vi "Heater_Safety.vi"   [LabVIEW 2010]
types:
  T1 = typedef "Ch_description_ADAM.ctl" = cluster{"Ch Name":string, "Type":T2, "Function":T3, "Ch State":T4, "Calibration type":T5, "A":dbl, "B":dbl, "C":dbl, "D":dbl, "Comments":string, "Address":T6, "String":string, "Duty":u16}
  T2 = typedef "Module_type_ADAM.ctl" = enum16{"4011", "4012", "4013", "4014", "4016", "4017", "4018", "4021", "4050", "4052", "4053", "4060", "4080", "5000", "5017", "5018", "5024", "5051", "5056", "5060", "6060", "Tracker", "WEST", "GILL", "JEM", "VICI", "Vaisala", "DRUCK", "Run VI Named:", "IR2100", "PPT", "Comparator", "VIRTUAL", "Hold Value", "Read A", "Read Ch", "Coded", "Client Info", "Web Client", "X10", "Test"}
  T3 = typedef "Function_ADAM.ctl" = enum16{"Analogue Input", "Digital Input", "Event counter", "Event rate", "Analogue Output", "Digital Output", "Relay Output"}
  T4 = typedef "Channel_State.ctl" = enum16{"On", "Off", "Always On", "Always Off"}
  T5 = typedef "Calib_type_ADAM.ctl" = enum16{"Raw", "Bx + A", "Cx^2 + Bx + A", "Dx^3 + Cx^2 + Bx + A", "In Band", "Hi-Tec Q", "Hi-Tec M_dot", "Text"}
  T6 = typedef "Address.ctl" = cluster{"Main":i32, "Ch.":i32, "Sub":i32, "Port Name":string}
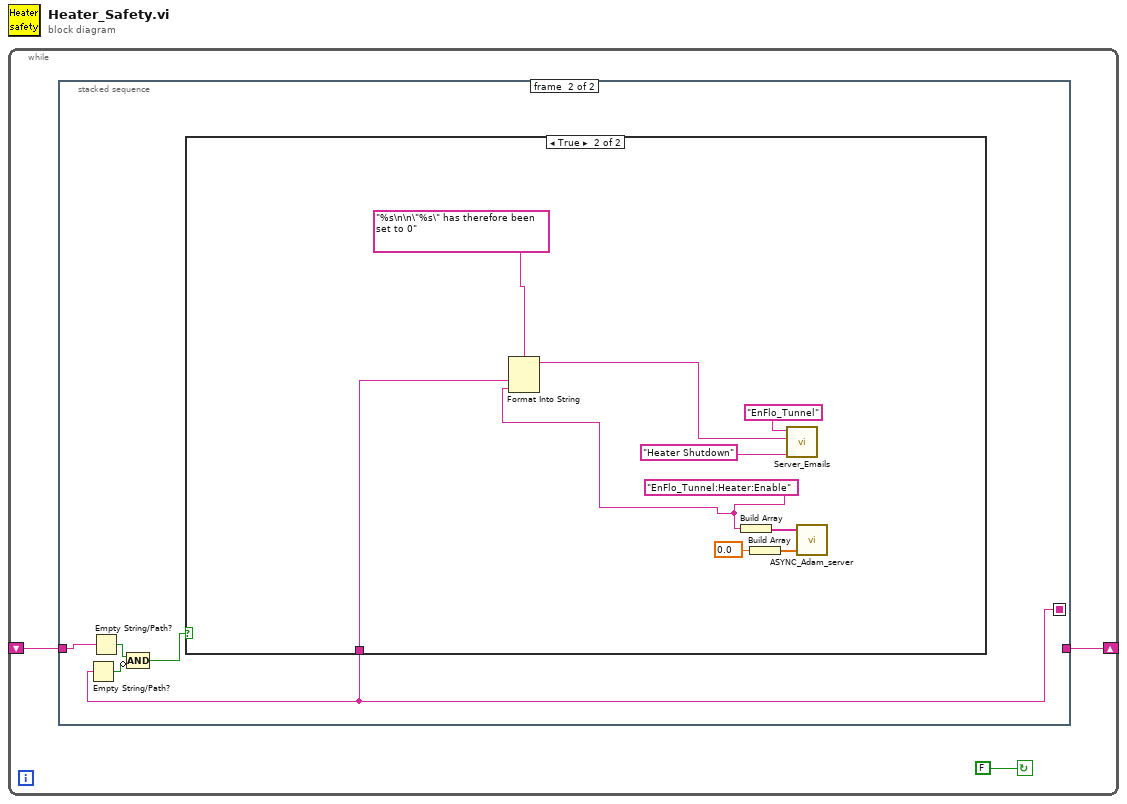
[diagram p0: block diagram]
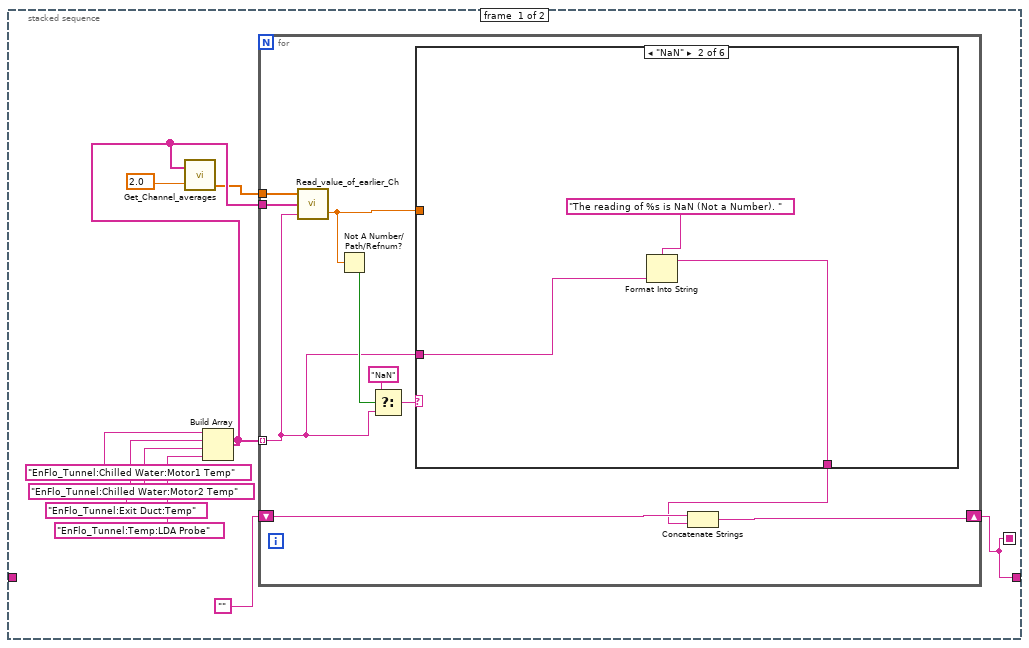
[diagram p2: hidden frame]
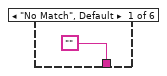
[diagram p3: hidden frame]
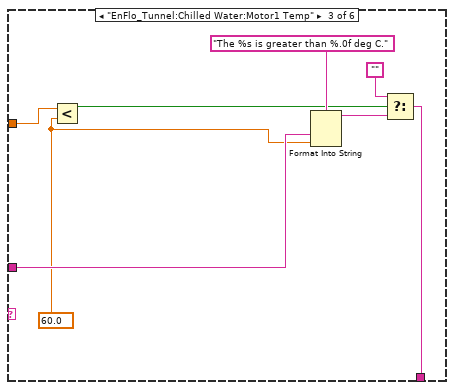
[diagram p4: hidden frame]
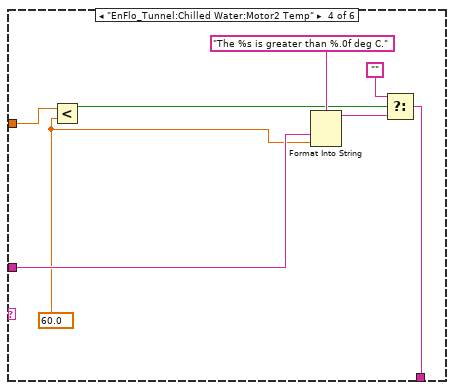
[diagram p5: hidden frame]
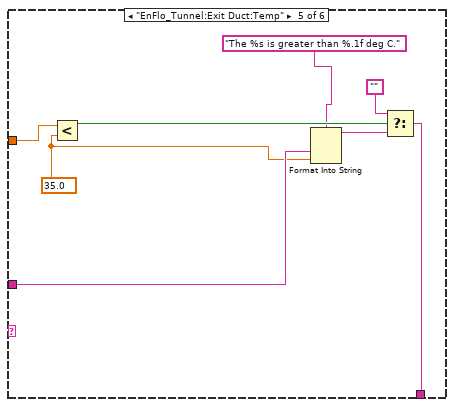
[diagram p6: hidden frame]
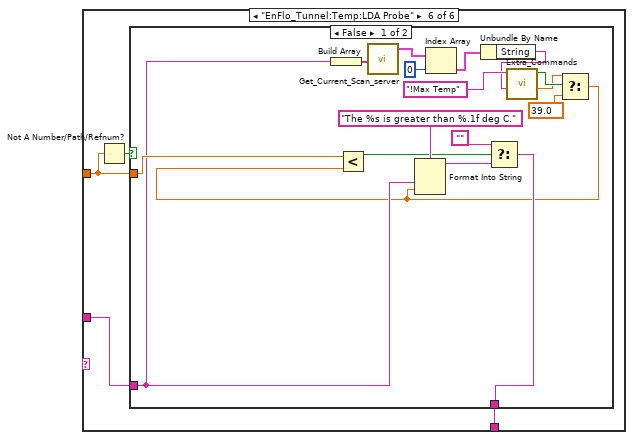
[diagram p7: hidden frame]
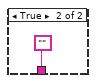
[diagram p8: hidden frame]
diagram:
  n1 = while {
    shift-left: _ -> [w1]
    shift-right: [w2] -> _
    stop <- FALSE continue-if-true
    n2 = stacked-sequence {
      seq-local: [w5 _] -> [_ w73]
      tunnel: [w5 _] -> w2
      tunnel: w1 -> [_ w77]
      frame #0 {
        n3 = Build Array("EnFlo_Tunnel:Chilled Water:Motor1 Temp", "EnFlo_Tunnel:Chilled Water:Motor2 Temp", "EnFlo_Tunnel:Exit Duct:Temp", "EnFlo_Tunnel:Temp:LDA Probe") -> (w9:string[])
        n4 = call "Get_Channel_averages.vi"("Desired Ch Names"=w9, "Averaging time (mins)"=2.0) -> ("number"=w6:dbl[])  [unwired: 1 in, 2 out]
        n5 = for {
          tunnel: w9 -> [w21]
          tunnel: w6 -> [w22]
          tunnel: w9 -> [w14] mode=indexing
          shift-right: [w19] -> w5
          shift-left: "" -> [w20]
          n6 = call "Read_value_of_earlier_Ch.vi"("Desired Ch to Read"=w14, "Ch names"=w21, "Present scan array"=w22) -> ("Value"=w17:dbl)  [unwired: 1 in, 1 out]
          n7 = Not A Number/Path/Refnum?(number/path/refnum=w17) -> (NaN/Path/Refnum?=w16:bool)
          n8 = Select(t="NaN", s=w16, f=w14) -> (s? t:f=w13:string)
          n9 = case shown="\"NaN\"" w13 {
            tunnel: w17 -> [_ _ w34 w42 w46 w52]
            tunnel: w14 -> [_ w24 w33 w41 w50 w54]
            tunnel: ["" w25 w27 w35 w47 w53] -> w18
            frame "No Match", Default {
            }
            frame "NaN" {
              n10 = Format Into String(format string="The reading of %s is NaN (Not a Number). " ("Format String"), w24) -> (resulting string=w25:string)  [unwired: 2 in, 1 out]
            }
            frame "EnFlo_Tunnel:Chilled Water:Motor1 Temp" {
              w32 = 60.0 ("y")
              n11 = Less?(x=w34, y=w32) -> (x < y?=w30:bool)
              n12 = Format Into String(format string="The %s is greater than %.0f deg C." ("Format String"), w33, w32) -> (resulting string=w29:string)  [unwired: 2 in, 1 out]
              n13 = Select(t="", s=w30, f=w29) -> (s? t:f=w27:string)
            }
            frame "EnFlo_Tunnel:Chilled Water:Motor2 Temp" {
              w40 = 60.0 ("y")
              n14 = Less?(x=w42, y=w40) -> (x < y?=w38:bool)
              n15 = Format Into String(format string="The %s is greater than %.0f deg C." ("Format String"), w41, w40) -> (resulting string=w37:string)  [unwired: 2 in, 1 out]
              n16 = Select(t="", s=w38, f=w37) -> (s? t:f=w35:string)
            }
            frame "EnFlo_Tunnel:Exit Duct:Temp" {
              w49 = 35.0 ("y")
              n17 = Less?(x=w46, y=w49) -> (x < y?=w48:bool)
              n18 = Format Into String(format string="The %s is greater than %.1f deg C." ("Format String"), w50, w49) -> (resulting string=w44:string)  [unwired: 2 in, 1 out]
              n19 = Select(t="", s=w48, f=w44) -> (s? t:f=w47:string)
            }
            frame "EnFlo_Tunnel:Temp:LDA Probe" {
              n20 = Not A Number/Path/Refnum?(number/path/refnum=w52) -> (NaN/Path/Refnum?=w51:bool)
              n21 = case shown="False" w51 {
                tunnel: w52 -> [w71 _]
                tunnel: w54 -> [w65 _]
                tunnel: [w66 ""] -> w53
                frame False {
                  n22 = Build Array(w65) -> (w64:string[])
                  n23 = call "Get_Current_Scan_server.vi"("Desired Channels"=w64) -> ("Ch Description Array"=w63:T1[])  [unwired: 2 out]
                  n24 = Index Array(array=w63, index=0 ("Index")) -> (element=w61:T1)
                  n25 = Unbundle By Name(w61) -> ("String"=w55:string)
                  n26 = call "Extra_Commands.vi"("String to Search"=w55, "Command"="!Max Temp") -> ("Numeric Value"=w58:dbl, "Command Found"=w59:bool)  [unwired: 1 in, 3 out]
                  n27 = Select(t=w58, s=w59, f=39.0) -> (s? t:f=w56:dbl)
                  n28 = Less?(x=w71, y=w56) -> (x < y?=w67:bool)
                  n29 = Format Into String(format string="The %s is greater than %.1f deg C." ("Format String"), w65, w56) -> (resulting string=w69:string)  [unwired: 2 in, 1 out]
                  n30 = Select(t="", s=w67, f=w69) -> (s? t:f=w66:string)
                }
                frame True {
                }
              }
            }
          }
          n31 = Concatenate Strings(w20, w18) -> (w19:string)
        }
      }
      frame #1 {
        n32 = Empty String/Path?(string/path=w73) -> (empty?=w75:bool)
        n33 = Empty String/Path?(string/path=w77) -> (empty?=w76:bool)
        n34 = Compound Arithmetic op=AND(w76, invert w75) -> (w74:bool)
        n35 = case shown="True" w74 {
          tunnel: w73 -> [_ w79]
          frame False {
          }
          frame True {
            w80 = "EnFlo_Tunnel:Heater:Enable"
            n36 = Format Into String(format string="%s\n\n\"%s\" has therefore been set to 0", w79, w80) -> (resulting string=w78:string)  [unwired: 2 in, 1 out]
            n37 = Build Array(w80) -> (w81:string[])
            n38 = Build Array(0.0) -> (w82:dbl[])
            n39 = call "Server_Emails.vi"("Client Name Contains"="EnFlo_Tunnel", "Message"=w78, "Subject"="Heater Shutdown" ("t")) -> ()  [unwired: 2 in, 3 out]
            n40 = call "ASYNC_Adam_server.vi"("Values"=w82, "Channel Names"=w81) -> ()  [unwired: 1 in, 3 out]
          }
        }
      }
    }
  }
